vi "5 Balls.vi"(10 "Where":string) -> ()   [LabVIEW 2019]
uses:
  TurretMode.ctl
  MotorsGlobal.vi
  JoysticksGlobal.vi
  StateMachine_5BallLoadingBay.ctl
panel:
  in  "PIDs":T1(tab)
  in  "Anda1_TimeLimit":dbl
  in  "Distance1":dbl
  in  "DelayAnda1":i32=300
  in  "Setpoint_CurvaEsq1":dbl
  in  "GainsCurvaEsq1":T2={"proportional gain (Kc)"=1.0, "integral time (Ti, min)"=0.01, "derivative time (Td, min)"=0.0} {"derivative time (Td, min)" format="%.3f"; "integral time (Ti, min)" format="%.3f"; "proportional gain (Kc)" format="%.3f"}
  in  "RangeCurvaEsq1":cluster{"output high":dbl, "output low":dbl}={"output high"=0.6, "output low"=-0.6} {"output low" format="%.2f"; "output high" format="%.2f"}
  in  "CurvaEsq1_TimeLimit":dbl
  in  "Distance2":dbl
  in  "Anda2_TimeLimit":dbl
  in  "DelayAnda2":i32=300
  in  "GainsCurvaDir2":T2={"proportional gain (Kc)"=1.0, "integral time (Ti, min)"=0.01, "derivative time (Td, min)"=0.0} {"derivative time (Td, min)" format="%.3f"; "integral time (Ti, min)" format="%.3f"; "proportional gain (Kc)" format="%.3f"}
  in  "RangeCurvaDir2":cluster{"output high":dbl, "output low":dbl}={"output high"=0.6, "output low"=-0.6} {"output low" format="%.2f"; "output high" format="%.2f"}
  in  "Setpoint_CurvaDir2":dbl
  in  "CurvaDir2_TimeLimit":dbl
  in  "Anda3_TimeLimit":dbl
  in  "DelayAnda3":i32=300
  in  "Distance3":dbl
  in  "GainsCurvaDir3":T2={"proportional gain (Kc)"=1.0, "integral time (Ti, min)"=0.01, "derivative time (Td, min)"=0.0} {"derivative time (Td, min)" format="%.3f"; "integral time (Ti, min)" format="%.3f"; "proportional gain (Kc)" format="%.3f"}
  in  "RangeCurvaDir3":cluster{"output high":dbl, "output low":dbl}={"output high"=0.6, "output low"=-0.6} {"output low" format="%.2f"; "output high" format="%.2f"}
  in  "Setpoint_CurvaDir3":dbl
  in  "CurvaDir3_TimeLimit":dbl
  in  "AlinhaLL_TimeLimit":dbl
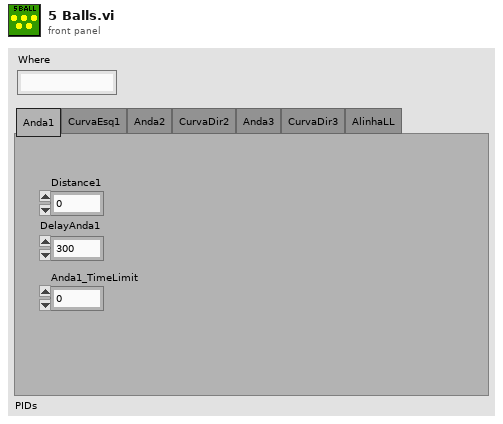
[diagram p1: front panel]
types:
  T1 = enum32{"Anda1", "CurvaEsq1", "Anda2", "CurvaDir2", "Anda3", "CurvaDir3", "AlinhaLL"}
  T2 = cluster{"proportional gain (Kc)":dbl, "integral time (Ti, min)":dbl, "derivative time (Td, min)":dbl}
  T3 = typedef "StateMachine_5BallLoadingBay.ctl" = enum16{"Standart", "Anda1", "CurvaEsq1", "Reset1", "Anda2", "CurvaDir2", "Reset2", "Anda3", "CurvaDir3", "AlinhaLL", "Atira"}
  T4 = typedef "TurretMode.ctl" = enum16{"Static", "Manual", "Automatic"}
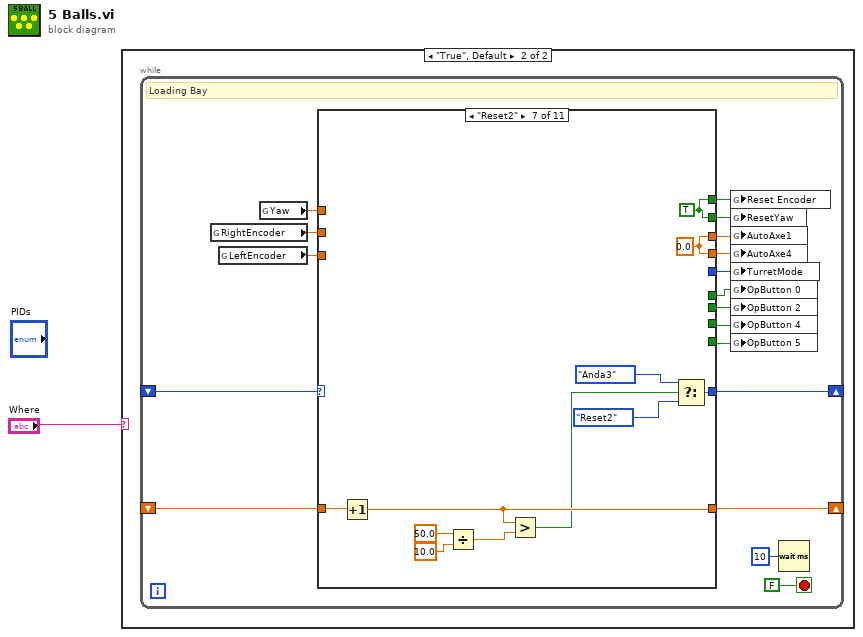
[diagram p0: block diagram]
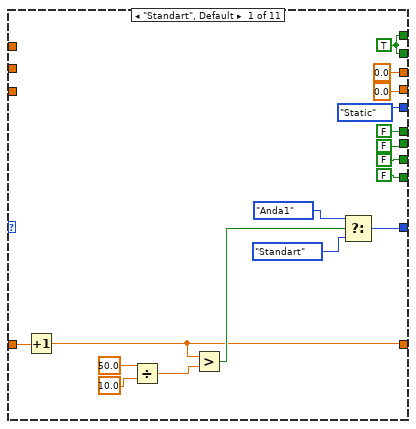
[diagram p3: hidden frame]
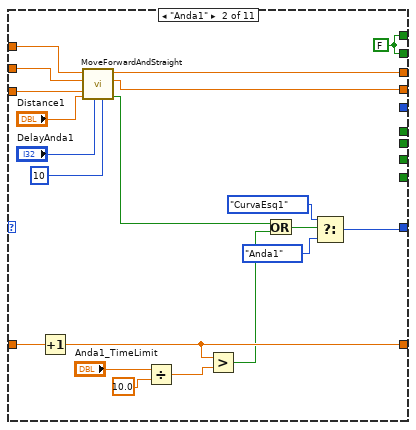
[diagram p4: hidden frame]
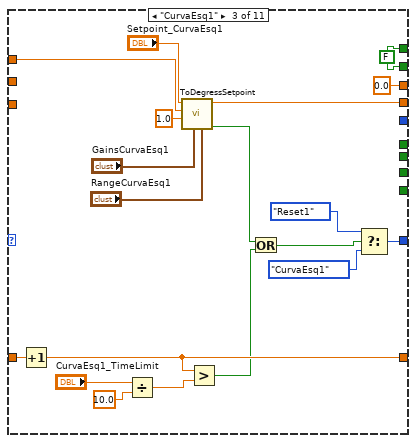
[diagram p5: hidden frame]
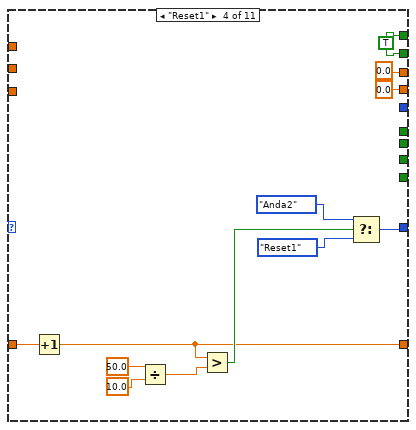
[diagram p6: hidden frame]
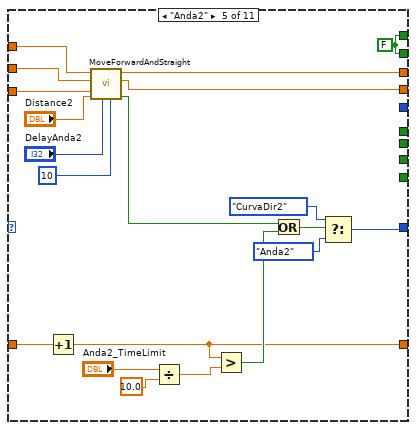
[diagram p7: hidden frame]
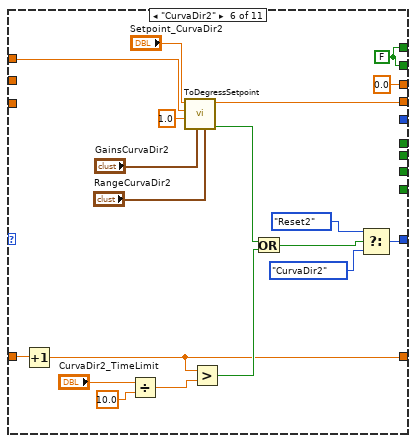
[diagram p8: hidden frame]
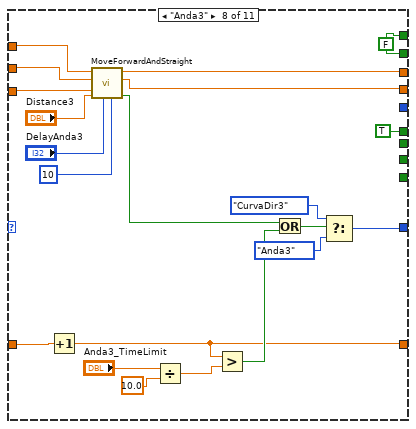
[diagram p9: hidden frame]
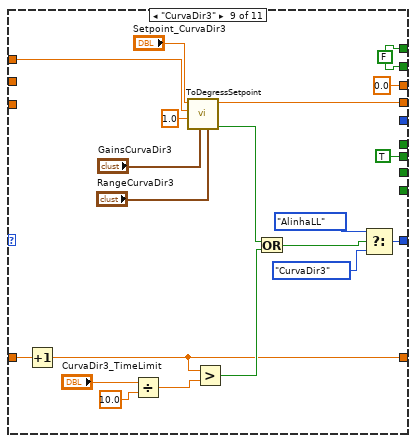
[diagram p10: hidden frame]
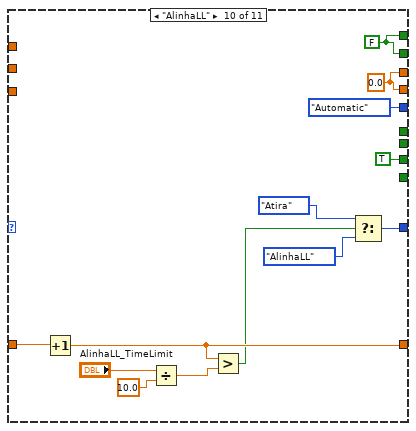
[diagram p11: hidden frame]
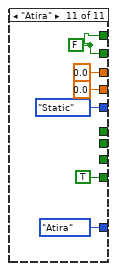
[diagram p12: hidden frame]
diagram:
  n1 = case shown="\"True\", Default" "Where" {
    frame "False" {
    }
    frame "True", Default {
      n2 = while {
        shift-right: [w7] -> _
        shift-left: _ -> [w19]
        shift-right: [w14] -> _
        shift-left: _ -> [w15]
        stop <- FALSE stop-if-true
        # "Loading Bay"
        n3 = global read "MotorsGlobal.vi" "RightEncoder"() -> (w17:dbl)
        n4 = global read "MotorsGlobal.vi" "LeftEncoder"() -> (w18:dbl)
        n5 = global read "MotorsGlobal.vi" "Yaw"() -> (w16:dbl)
        n6 = case shown="\"Reset2\"" w19 {
          tunnel: w18 -> [_ w56 _ _ w96 _ _ w145 _ _ _]
          tunnel: w17 -> [_ w55 _ _ w97 _ _ w146 _ _ _]
          tunnel: w16 -> [_ w54 w75 _ w98 w113 _ w147 w162 _ _]
          tunnel: w15 -> [w31 w49 w66 w83 w95 w116 w134 w139 w166 w185 _]
          tunnel: [w27 w47 w65 w82 w94 w115 w133 w138 w165 w184 _] -> w14
          tunnel: [0.0 ("Direction") w42 w72 0.0 ("Direction") w93 w114 w127 w144 w163 w179 0.0 ("Output")] -> w11
          tunnel: [0.0 ("Trottle") w41 0.0 ("Trottle") 0.0 ("Trottle") w92 0.0 ("Trottle") w127 w143 0.0 ("Trottle") w179 0.0 ("Trottle")] -> w10
          tunnel: [w34 w40 w61 w81 w91 w112 w128 w140 w160 w190 w194] -> w9
          tunnel: [w34 w40 w61 w81 w91 w112 w128 w140 w160 w190 w194] -> w8
          tunnel: [w29 w39 w60 w78 w90 w111 w131 w142 w164 w183 StateMachine_5BallLoadingBay."Atira"] -> w7
          tunnel: [TurretMode."Static" ("TurretMode") _ _ _ _ _ _ _ _ TurretMode."Automatic" ("TurretMode") TurretMode."Static" ("TurretMode")] -> w6
          tunnel: [FALSE ("OpButton 4") _ _ _ _ _ _ _ _ TRUE ("OpButton 4") _] -> w5
          tunnel: [FALSE ("OpButton 5") _ _ _ _ _ _ _ _ _ TRUE ("OpButton 5")] -> w4
          tunnel: [FALSE ("OpButton 5") _ _ _ _ _ _ _ TRUE ("OpButton 5") _ _] -> w3
          tunnel: [FALSE ("OpButton 4") _ _ _ _ _ _ TRUE ("OpButton 4") _ _ _] -> w2
          frame "Standart", Default {
            w34 = TRUE
            n7 = Increment(x=w31) -> (x+1=w27:dbl)
            n8 = Divide(x=50.0, y=10.0) -> (x/y=w33:dbl)
            n9 = Greater?(x=w27, y=w33) -> (0:w28:bool)
            n10 = Select(t=StateMachine_5BallLoadingBay."Anda1", s=w28, f=StateMachine_5BallLoadingBay."Standart") -> (s? t:f=w29:T3)
          }
          frame "Anda1" {
            w40 = FALSE
            n11 = Increment(x=w49) -> (x+1=w47:dbl)
            n12 = call "MoveForwardAndStraight.vi"("Loop Timer"=10, "Time to stop"="DelayAnda1", "Distance"="Distance1", "Encoder Left"=w56, "Encoder Right"=w55, "Yaw"=w54) -> ("Finished distance"=w50:bool, "Direction"=w42:dbl, "Trottle"=w41:dbl)  [unwired: 2 in, 1 out]
            n13 = Divide(x="Anda1_TimeLimit", y=10.0) -> (x/y=w48:dbl)
            n14 = Greater?(x=w47, y=w48) -> (0:w46:bool)
            n15 = Or(x=w50, y=w46) -> (x .or. y?=w45:bool)
            n16 = Select(t=StateMachine_5BallLoadingBay."CurvaEsq1", s=w45, f=StateMachine_5BallLoadingBay."Anda1") -> (s? t:f=w39:T3)
          }
          frame "CurvaEsq1" {
            w61 = FALSE
            n17 = Increment(x=w66) -> (x+1=w65:dbl)
            n18 = Divide(x="CurvaEsq1_TimeLimit", y=10.0) -> (x/y=w68:dbl)
            n19 = call "ToDegressSetpoint.vi"("Range"="RangeCurvaEsq1", "Gains"="GainsCurvaEsq1", "Precision"=1.0, "Yaw"=w75, "Setpoint (degress)"="Setpoint_CurvaEsq1") -> ("Finished?"=w62:bool, "Output"=w72:dbl)  [unwired: 5 in]
            n20 = Greater?(x=w65, y=w68) -> (0:w63:bool)
            n21 = Or(x=w62, y=w63) -> (x .or. y?=w64:bool)
            n22 = Select(t=StateMachine_5BallLoadingBay."Reset1", s=w64, f=StateMachine_5BallLoadingBay."CurvaEsq1") -> (s? t:f=w60:T3)
          }
          frame "Reset1" {
            w81 = TRUE
            n23 = Increment(x=w83) -> (x+1=w82:dbl)
            n24 = Divide(x=50.0, y=10.0) -> (x/y=w87:dbl)
            n25 = Greater?(x=w82, y=w87) -> (0:w84:bool)
            n26 = Select(t=StateMachine_5BallLoadingBay."Anda2", s=w84, f=StateMachine_5BallLoadingBay."Reset1") -> (s? t:f=w78:T3)
          }
          frame "Anda2" {
            w91 = FALSE
            n27 = Increment(x=w95) -> (x+1=w94:dbl)
            n28 = call "MoveForwardAndStraight.vi"("Loop Timer"=10, "Time to stop"="DelayAnda2", "Distance"="Distance2", "Encoder Left"=w96, "Encoder Right"=w97, "Yaw"=w98) -> ("Finished distance"=w104:bool, "Direction"=w93:dbl, "Trottle"=w92:dbl)  [unwired: 2 in, 1 out]
            n29 = Divide(x="Anda2_TimeLimit", y=10.0) -> (x/y=w103:dbl)
            n30 = Greater?(x=w94, y=w103) -> (0:w102:bool)
            n31 = Or(x=w104, y=w102) -> (x .or. y?=w101:bool)
            n32 = Select(t=StateMachine_5BallLoadingBay."CurvaDir2", s=w101, f=StateMachine_5BallLoadingBay."Anda2") -> (s? t:f=w90:T3)
          }
          frame "CurvaDir2" {
            w112 = FALSE
            n33 = Increment(x=w116) -> (x+1=w115:dbl)
            n34 = Divide(x="CurvaDir2_TimeLimit", y=10.0) -> (x/y=w121:dbl)
            n35 = call "ToDegressSetpoint.vi"("Range"="RangeCurvaDir2", "Gains"="GainsCurvaDir2", "Precision"=1.0, "Yaw"=w113, "Setpoint (degress)"="Setpoint_CurvaDir2") -> ("Finished?"=w117:bool, "Output"=w114:dbl)  [unwired: 5 in]
            n36 = Greater?(x=w115, y=w121) -> (0:w118:bool)
            n37 = Or(x=w117, y=w118) -> (x .or. y?=w119:bool)
            n38 = Select(t=StateMachine_5BallLoadingBay."Reset2", s=w119, f=StateMachine_5BallLoadingBay."CurvaDir2") -> (s? t:f=w111:T3)
          }
          frame "Reset2" {
            w127 = 0.0 ("Trottle")
            w128 = TRUE
            n39 = Increment(x=w134) -> (x+1=w133:dbl)
            n40 = Divide(x=50.0, y=10.0) -> (x/y=w136:dbl)
            n41 = Greater?(x=w133, y=w136) -> (0:w132:bool)
            n42 = Select(t=StateMachine_5BallLoadingBay."Anda3", s=w132, f=StateMachine_5BallLoadingBay."Reset2") -> (s? t:f=w131:T3)
          }
          frame "Anda3" {
            w140 = FALSE
            n43 = Increment(x=w139) -> (x+1=w138:dbl)
            n44 = call "MoveForwardAndStraight.vi"("Loop Timer"=10, "Time to stop"="DelayAnda3", "Distance"="Distance3", "Encoder Left"=w145, "Encoder Right"=w146, "Yaw"=w147) -> ("Finished distance"=w155:bool, "Direction"=w144:dbl, "Trottle"=w143:dbl)  [unwired: 2 in, 1 out]
            n45 = Divide(x="Anda3_TimeLimit", y=10.0) -> (x/y=w154:dbl)
            n46 = Greater?(x=w138, y=w154) -> (0:w153:bool)
            n47 = Or(x=w155, y=w153) -> (x .or. y?=w152:bool)
            n48 = Select(t=StateMachine_5BallLoadingBay."CurvaDir3", s=w152, f=StateMachine_5BallLoadingBay."Anda3") -> (s? t:f=w142:T3)
          }
          frame "CurvaDir3" {
            w160 = FALSE
            n49 = Increment(x=w166) -> (x+1=w165:dbl)
            n50 = Divide(x="CurvaDir3_TimeLimit", y=10.0) -> (x/y=w173:dbl)
            n51 = call "ToDegressSetpoint.vi"("Range"="RangeCurvaDir3", "Gains"="GainsCurvaDir3", "Precision"=1.0, "Yaw"=w162, "Setpoint (degress)"="Setpoint_CurvaDir3") -> ("Finished?"=w169:bool, "Output"=w163:dbl)  [unwired: 5 in]
            n52 = Greater?(x=w165, y=w173) -> (0:w170:bool)
            n53 = Or(x=w169, y=w170) -> (x .or. y?=w171:bool)
            n54 = Select(t=StateMachine_5BallLoadingBay."AlinhaLL", s=w171, f=StateMachine_5BallLoadingBay."CurvaDir3") -> (s? t:f=w164:T3)
          }
          frame "AlinhaLL" {
            w179 = 0.0 ("Trottle")
            w190 = FALSE
            n55 = Increment(x=w185) -> (x+1=w184:dbl)
            n56 = Divide(x="AlinhaLL_TimeLimit", y=10.0) -> (x/y=w187:dbl)
            n57 = Greater?(x=w184, y=w187) -> (0:w180:bool)
            n58 = Select(t=StateMachine_5BallLoadingBay."Atira", s=w180, f=StateMachine_5BallLoadingBay."AlinhaLL") -> (s? t:f=w183:T3)
          }
          frame "Atira" {
            w194 = FALSE
          }
        }
        n59 = global write "MotorsGlobal.vi" "Reset Encoder"(w9) -> ()
        n60 = global write "MotorsGlobal.vi" "ResetYaw"(w8) -> ()
        n61 = global write "JoysticksGlobal.vi" "AutoAxe1"(w10) -> ()
        n62 = global write "JoysticksGlobal.vi" "AutoAxe4"(w11) -> ()
        n63 = global write "MotorsGlobal.vi" "TurretMode"(w6) -> ()
        n64 = global write "JoysticksGlobal.vi" "OpButton 0"(w2) -> ()
        n65 = global write "JoysticksGlobal.vi" "OpButton 2"(w3) -> ()
        n66 = global write "JoysticksGlobal.vi" "OpButton 4"(w5) -> ()
        n67 = global write "JoysticksGlobal.vi" "OpButton 5"(w4) -> ()
        n68 = Wait (ms)(milliseconds to wait=u32 10) -> ()  [unwired: 1 out]
      }
    }
  }
